vi "BuildMenu.vi"(8 "error in (no error)":errorcluster, 10 "menu reference":refnum<k9>, 11 "DAQ_Module in":refnum<class "DAQ_Module.lvclass">) -> (0 "error out":errorcluster, 3 "DAQ_Module out":refnum<class "DAQ_Module.lvclass">)   [LabVIEW 2025, in "DAQ_Module.lvlib" / "DAQ_Module.lvclass"]
uses:
  DAQ_Module.lvclass
  DAQ_Module.lvclass/DAQ_Module.ctl
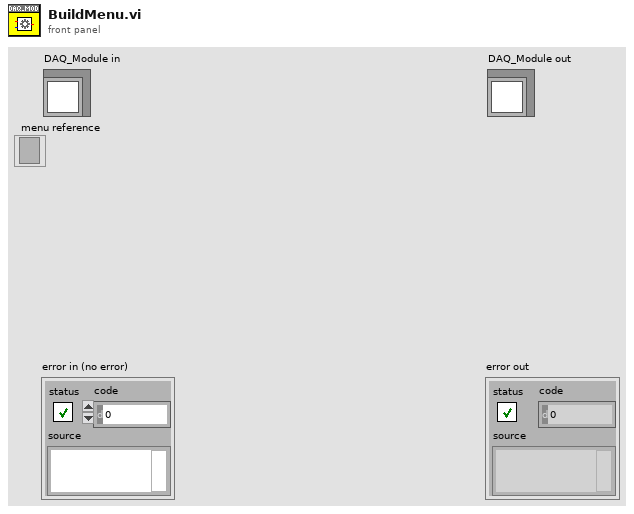
[diagram p1: front panel]
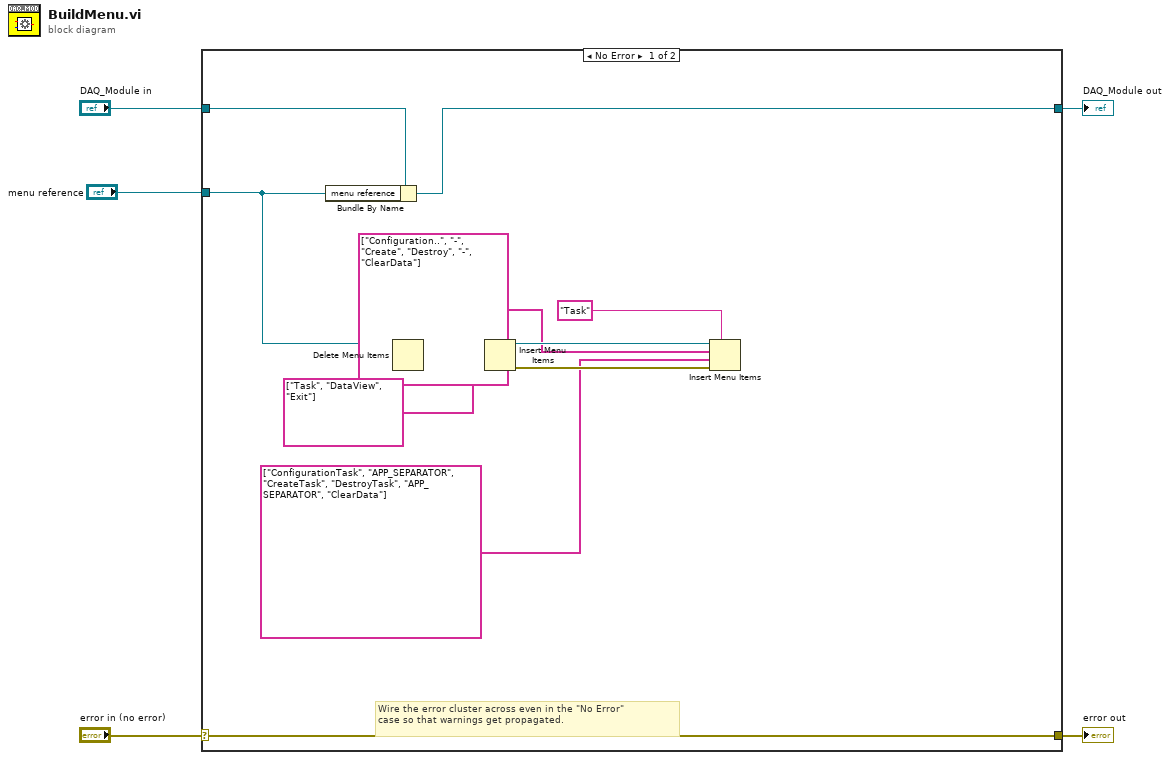
[diagram p0: block diagram]
diagram:
  n1 = case shown="No Error" "error in (no error)" {
    selector: "error in (no error)" -> [w17 w19]
    tunnel: [w17 w19] -> w4
    tunnel: [w15 w18] -> w2
    tunnel: "DAQ_Module in" -> [w16 w18]
    tunnel: "menu reference" -> [w14 _]
    frame No Error {
      # "Wire the error cluster across even in the \"No Error\"\ncase so that warnings get propagated."
      n2 = Bundle By Name(cluster=w16, "menu reference"=w14) -> (w15:refnum<class "DAQ_Module.lvclass">)
      n3 = Delete Menu Items(9:w14) -> (0:w7:errorcluster, 3:w8:refnum<k9>)  [unwired: 3 in]
      n4 = Insert Menu Items(6:w7, 7:string[] ["Task", "DataView", "Exit"], 9:w8) -> (0:w11:errorcluster, 3:w12:refnum<k9>)  [unwired: 3 in, 1 out]
      n5 = Insert Menu Items(5:"Task", 6:w11, 7:string[] ["ConfigurationTask", "APP_SEPARATOR", "CreateTask", "DestroyTask", "APP_SEPARATOR", "ClearData"], 8:string[] ["Configuration..", "-", "Create", "Destroy", "-", "ClearData"], 9:w12) -> ()  [unwired: 1 in, 3 out]
    }
    frame Error {
    }
  }
  "error out" <- w4
  "DAQ_Module out" <- w2
